vi "SaveImageData.vi"(0 "object in":refnum<class "Experiment2.lvclass">, 2 "Timestamps":dbl[](array[numeric]), 3 "Filenames":path[](array[path]), 5 "error in (no error)":errorcluster) -> (14 "object out":refnum<class "Experiment2.lvclass">, 19 "error out":errorcluster)   [LabVIEW 2021, in "Experiment2.lvclass"]
uses:
  Experiment2.lvclass
  Experiment2.lvclass/Experiment2.ctl
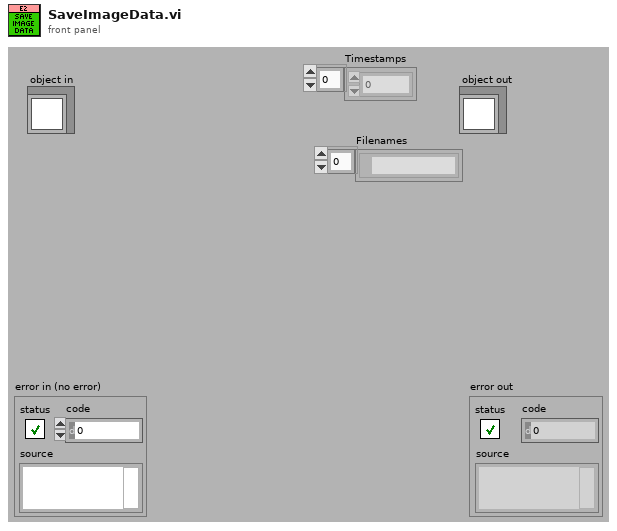
[diagram p1: front panel]
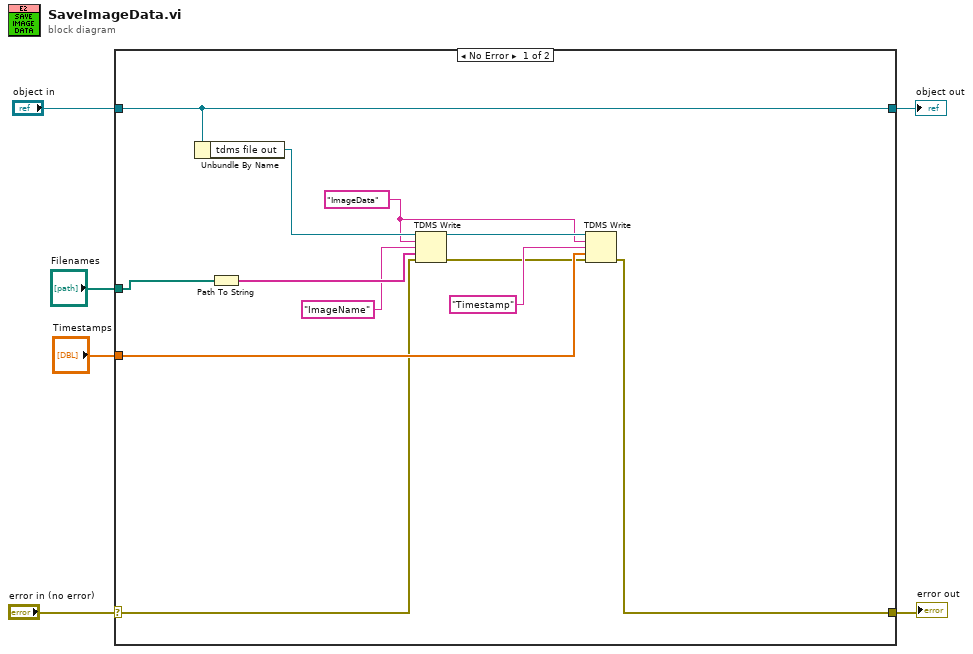
[diagram p0: block diagram]
diagram:
  n1 = case shown="No Error" "error in (no error)" {
    selector: "error in (no error)" -> [w8 w20]
    tunnel: [w7 w20] -> w5
    tunnel: [w18 w19] -> w3
    tunnel: "object in" -> [w18 w19]
    tunnel: "Filenames" -> [w16 _]
    tunnel: "Timestamps" -> [w11 _]
    frame No Error {
      w10 = "ImageData" ("group name in (Untitled)")
      n2 = Unbundle By Name(w18) -> ("tdms file out"=w17:refnum<k34>)
      n3 = Path To String(path=w16) -> (string=w15:string[])
      n4 = TDMS Write(0:w17, 5:w10, 7:"ImageName" ("group name in (Untitled)"), 9:w15, 11:w8) -> (4:w13:refnum<k34>, 15:w9:errorcluster)  [unwired: 1 in, 2 out]
      n5 = TDMS Write(0:w13, 5:w10, 7:"Timestamp" ("group name in (Untitled)"), 9:w11, 11:w9) -> (15:w7:errorcluster)  [unwired: 1 in, 3 out]
    }
    frame Error {
    }
  }
  "error out" <- w5
  "object out" <- w3
